vi "五参数水样测试.vi"(11 "启动参数":T1={"测量模式"=enum."水样测试", "数据标记表"="N", "测量时间"=3.0}) -> ()   [LabVIEW 2016, in "斯坦道仪器.lvlib"]
uses:
  PLC/PLC.lvlib
panel:
  out "枚举":T2(ring)
  out "状态":string
  out "数值":i32
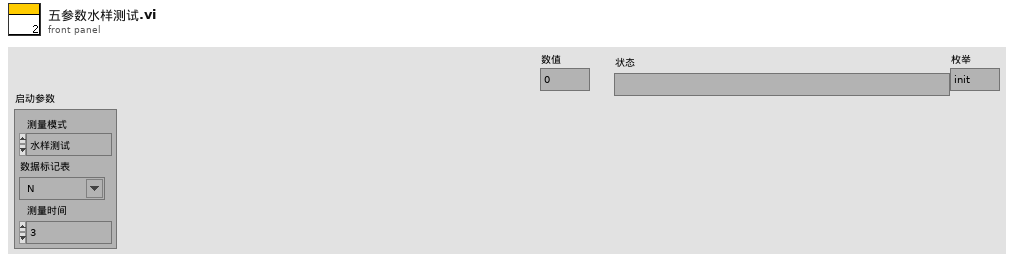
[diagram p1: front panel]
types:
  T1 = cluster{"测量模式":enum16{"待机", "水样测试", "标样核查", "零点核查", "跨度核查", "空白测试", "平行样测试", "加标回收", "空白校准", "标样校准", "初始化（清洗）"}, "数据标记表":string, "测量时间":dbl}
  T2 = enum16{"init", "开机", "启动测量", "读取测量值", "存储数据", "关闭测量", "关机", "结束"}
  T3 = cluster{"时间标识":timestamp, "设备":string, "日志信息":string, "流程参数":string}
  T4 = cluster{"starting address":u16, "holding register value":u16}
  T5 = enum16{"idle", "init", "读状态", "读参数", "多个写入", "单个写入", "线圈写入"}
  T6 = enum16{"待机", "水样测试", "标样核查", "零点核查", "跨度核查", "空白测试", "平行样测试", "加标回收", "空白校准", "标样校准", "初始化（清洗）"}
  T7 = cluster{"水温":dbl, "pH":dbl, "DO":dbl, "Cond":dbl, "Turb":dbl, "叶绿素":dbl, "藻密度":dbl, "蓝绿藻":dbl, "ORP":dbl, "NH3N":dbl}
  T8 = cluster{"数据标记表":string, "测量模式":enum16{"待机", "水样测试", "标样核查", "零点核查", "跨度核查", "空白测试", "平行样测试", "加标回收", "空白校准", "标样校准", "初始化（清洗）"}, "database":string}
  T9 = cluster{"因子编码":string, "单位":string, "标样参考值":sgl, "水样数据时间":timestamp, "水样实测值":sgl, "水样数据标识":string, "K":sgl, "B":sgl, "T":sgl, "H":sgl, "水深":sgl}
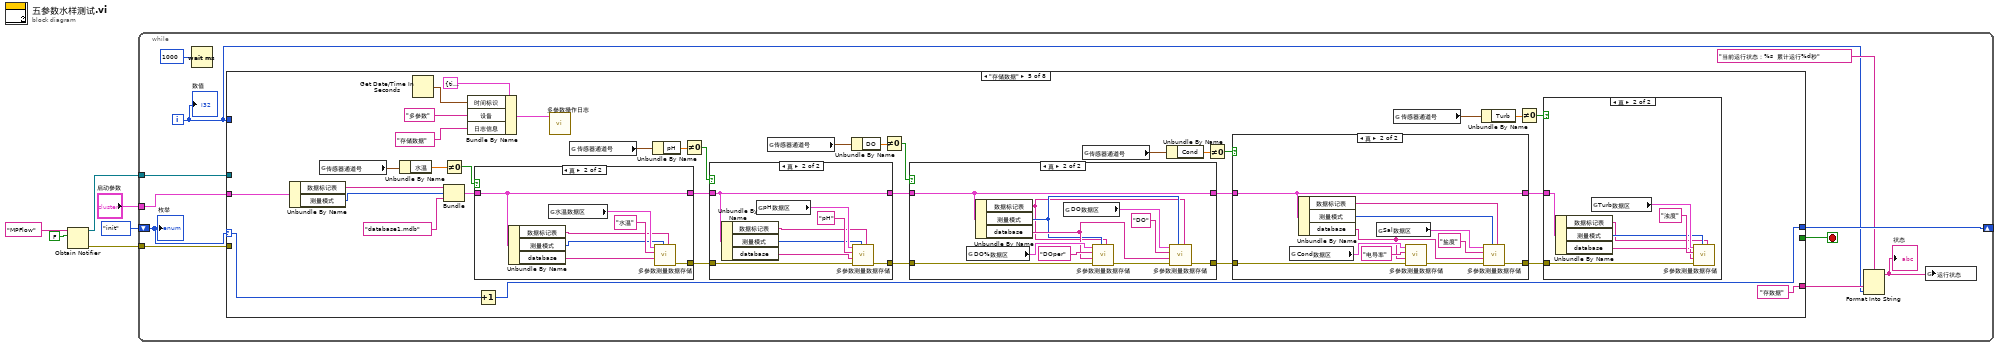
[diagram p0: block diagram]
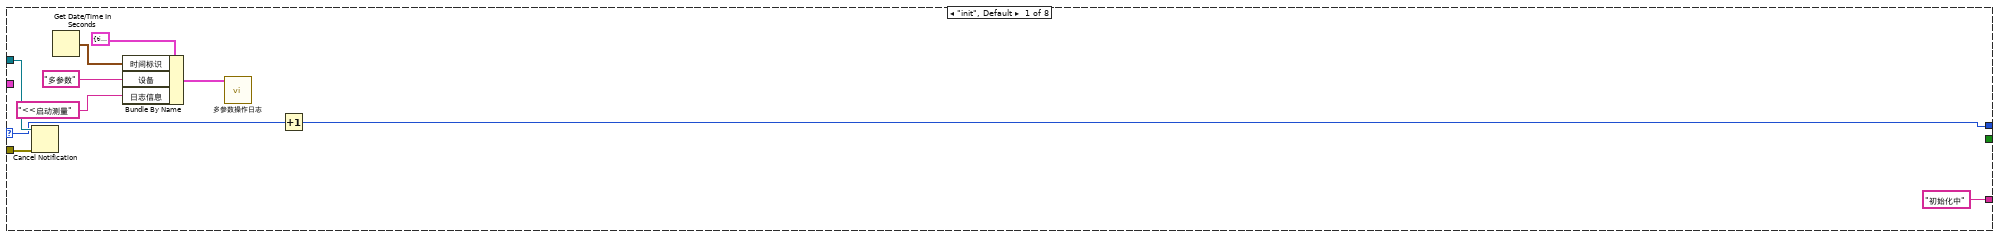
[diagram p2: hidden frame]
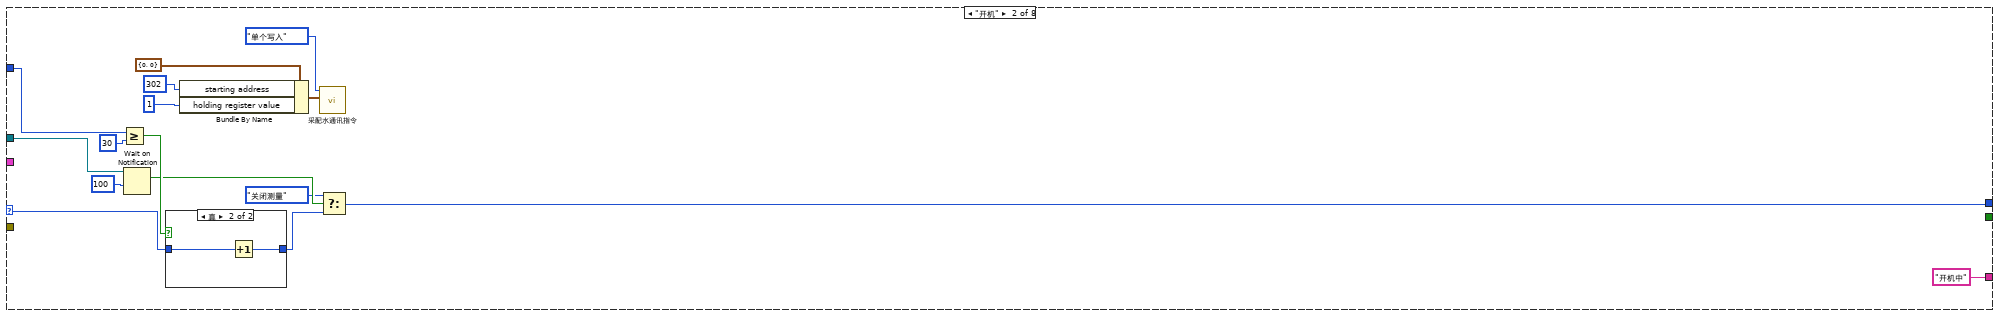
[diagram p3: hidden frame]
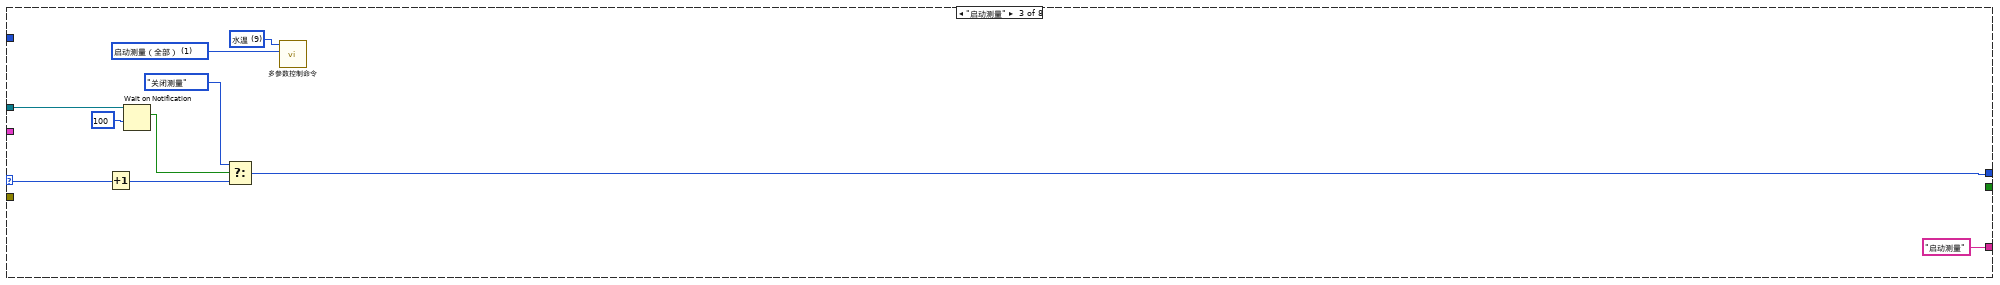
[diagram p5: hidden frame]
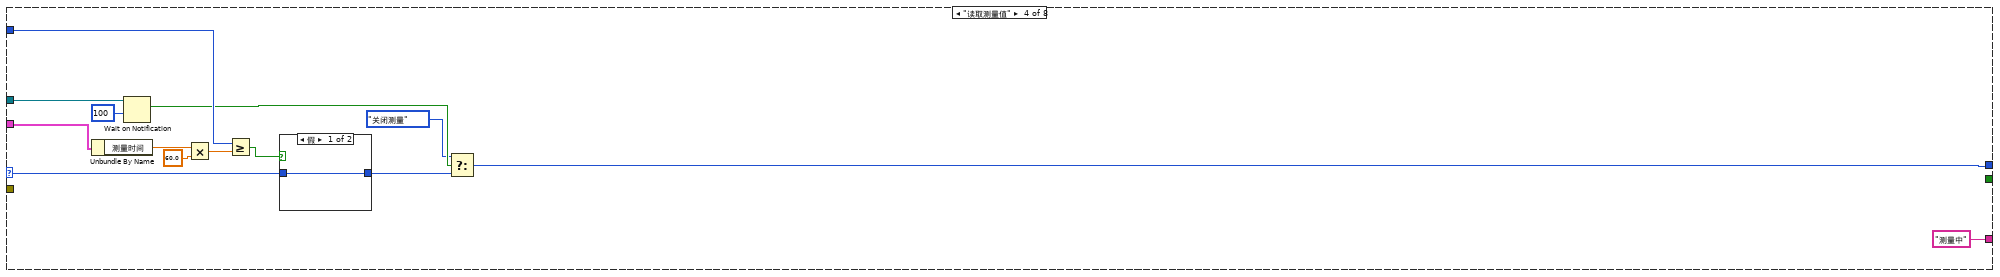
[diagram p6: hidden frame]
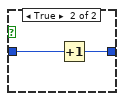
[diagram p7: hidden frame]
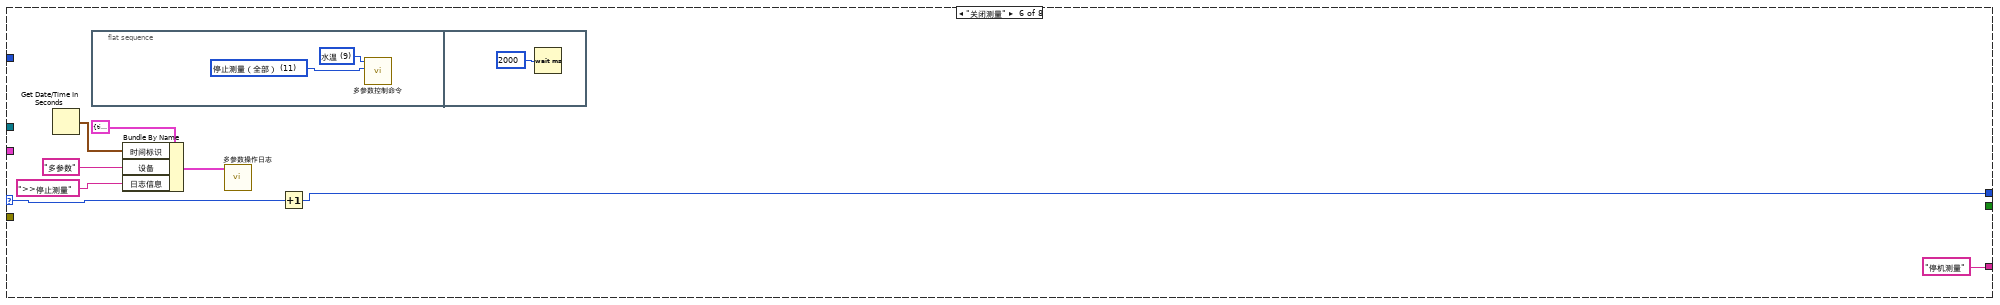
[diagram p13: hidden frame]
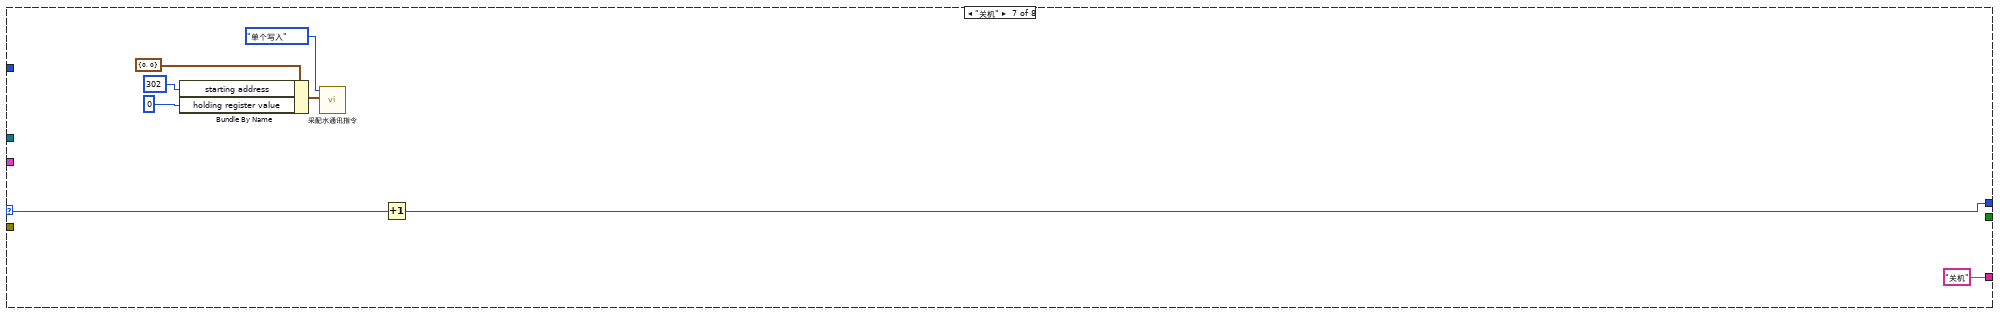
[diagram p14: hidden frame]
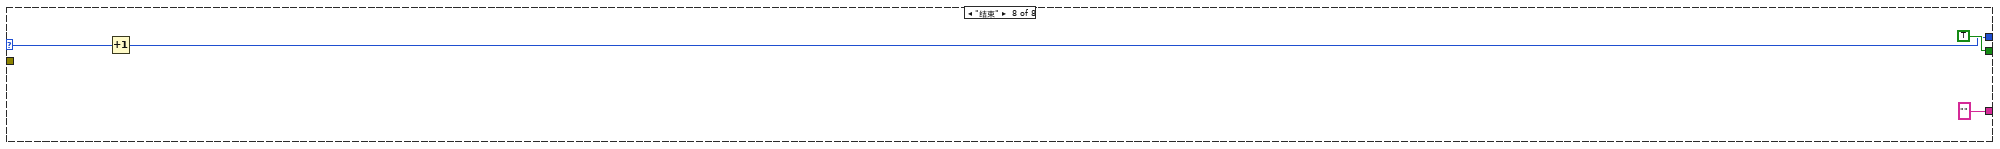
[diagram p15: hidden frame]
diagram:
  n1 = Obtain Notifier(name (unnamed)="MPFlow" ("名称（未命名）"), notification data type=FALSE) -> (notifier out=w3:refnum<notifier>, error out=w2:errorcluster)  [unwired: 2 in, 1 out]
  n2 = while {
    shift-right: [w13] -> _
    shift-left: T2."init" ("枚举") -> [w17]
    tunnel: w3 -> [w15]
    tunnel: w2 -> [w14]
    tunnel: "启动参数" -> [w7]
    i -> [w9]
    stop <- w16 stop-if-true
    n3 = Wait (ms)(milliseconds to wait=u32 1000 ("等待时间（毫秒）")) -> ()  [unwired: 1 out]
    n4 = case shown="\"存储数据\"" w17 {
      selector: w17 -> [w25 w38 w56 w69 w109 w165 w171 w179]
      tunnel: [_ _ _ _ _ _ _ TRUE] -> w16
      tunnel: w15 -> [w27 w33 w55 w66 _ _ _ _]
      tunnel: w14 -> [w26 _ _ _ _ _ _ _]
      tunnel: [w24 w31 w52 w64 w108 w164 w170 w178] -> w13
      tunnel: w9 -> [_ w37 _ w70 _ _ _ _]
      tunnel: ["初始化中" ("状态") "开机中" ("状态") "启动测量" ("状态") "测量中" ("状态") "存数据" ("状态") "停机测量" ("状态") "关机" ("状态") "" ("状态")] -> w10
      tunnel: w7 -> [_ _ _ w60 w106 _ _ _]
      frame "init", Default {
        n5 = Cancel Notification(0:w27, 3:w26) -> ()  [unwired: 3 out]
        n6 = Get Date/Time In Seconds() -> (seconds since 1Jan1904=w21:timestamp)
        n7 = Bundle By Name(cluster=T3 {"时间标识"=timestamp(0 s since 1904-01-01), "设备"="", "日志信息"="", "流程参数"=""} ("data in"), "时间标识"=w21, "设备"="多参数", "日志信息"="<<启动测量") -> (w20:T3)
        n8 = call "多参数操作日志.vi"("data in"=w20) -> ()  [unwired: 10 in, 1 out]
        n9 = Increment(x=w25) -> (x+1=w24:T2)
      }
      frame "开机" {
        n10 = Greater Or Equal?(x=w37, y=30) -> (x >= y?=w35:bool)
        n11 = Wait on Notification(notifier=w33, timeout in ms (-1)=100 ("超时毫秒(-1)")) -> (notification=w34:bool)  [unwired: 2 in, 3 out]
        n12 = case shown="真" w35 {
          tunnel: w38 -> [w44 w46]
          tunnel: [w44 w45] -> w32
          frame False {
          }
          frame True {
            n13 = Increment(x=w46) -> (x+1=w45:T2)
          }
        }
        n14 = Bundle By Name(cluster=T4 {"starting address"=0, "holding register value"=0}, "starting address"=u16 302, "holding register value"=u16 1) -> (w41:T4)
        n15 = call "采配水通讯指令.vi"("数据"=w41, "命令"=T5."单个写入") -> ()  [unwired: 10 in]
        n16 = Select(t=T2."关闭测量" ("枚举"), s=w34, f=w32) -> (s? t:f=w31:T2)
      }
      frame "启动测量" {
        w47 = u16 1 items=["启动测量（全部）"=1, "初始化（清洗）"=10, "停止测量（全部）"=11, "校时"=13, "启动测量（单个传感器）"=19, "停止测量（单个传感器）"=20] ("控制命令")
        w48 = u16 9 items=["氨氮"=3, "水温"=9, "pH值"=10, "溶解氧"=11, "电导率"=12, "浊度"=13, "叶绿素a"=14, "藻密度"=15, "蓝绿藻"=16, "氧化还原电位"=17, "溶解氧%"=18, "盐度"=19] ("站号")
        n17 = Increment(x=w56) -> (x+1=w53:T2)
        n18 = Wait on Notification(notifier=w55, timeout in ms (-1)=100 ("超时毫秒(-1)")) -> (notification=w54:bool)  [unwired: 2 in, 3 out]
        n19 = Select(t=T2."关闭测量" ("枚举"), s=w54, f=w53) -> (s? t:f=w52:T2)
        n20 = call "多参数控制命令.vi"("控制命令"=w47, "站号"=w48) -> ()  [unwired: 9 in, 1 out]
      }
      frame "读取测量值" {
        n21 = Unbundle By Name(w60) -> ("测量时间"=w59:dbl)
        n22 = Wait on Notification(notifier=w66, timeout in ms (-1)=100 ("超时毫秒(-1)")) -> (notification=w67:bool)  [unwired: 2 in, 3 out]
        n23 = Multiply(x=w59, y=60.0) -> (x*y=w57:dbl)
        n24 = Greater Or Equal?(x=w70, y=w57) -> (x >= y?=w68:bool)
        n25 = case shown="假" w68 {
          tunnel: w69 -> [w71 w73]
          tunnel: [w71 w72] -> w65
          frame False {
          }
          frame True {
            n26 = Increment(x=w73) -> (x+1=w72:T2)
          }
        }
        n27 = Select(t=T2."关闭测量" ("枚举"), s=w67, f=w65) -> (s? t:f=w64:T2)
      }
      frame "存储数据" {
        n28 = Unbundle By Name(w106) -> ("数据标记表"=w85:string, "测量模式"=w84:T6)
        n29 = global read "多参数全局变量.vi" "传感器通道号"() -> (w101:T7)
        n30 = Unbundle By Name(w101) -> ("水温"=w100:dbl)
        n31 = Get Date/Time In Seconds() -> (seconds since 1Jan1904=w77:timestamp)
        n32 = Not Equal To 0?(x=w100) -> (x != 0?=w99:bool)
        n33 = Bundle("数据标记表"=w85, "测量模式"=w84, "database"="database1.mdb") -> (w83:T8)  [unwired: 1 in]
        n34 = Bundle By Name(cluster=T3 {"时间标识"=timestamp(0 s since 1904-01-01), "设备"="", "日志信息"="", "流程参数"=""} ("data in"), "时间标识"=w77, "设备"="多参数", "日志信息"="存储数据") -> (w76:T3)
        n35 = case shown="真" w99 {
          tunnel: [_ w155] -> w105
          tunnel: w83 -> [w150 w154]
          tunnel: [w150 w154] -> w82
          frame False {
          }
          frame True {
            n36 = Unbundle By Name(w154) -> ("数据标记表"=w153:string, "测量模式"=w152:T6, "database"=w151:string)
            n37 = global read "多参数全局变量.vi" "水温数据区"() -> (w157:T9)
            n38 = call "多参数测量数据存储.vi"("数据标记表"=w153, "测量模式"=w152, "database"=w151, "table输入"="水温", "data in"=w157) -> ("error out"=w155:errorcluster)  [unwired: 6 in]
          }
        }
        n39 = Increment(x=w109) -> (x+1=w108:T2)
        n40 = call "多参数操作日志.vi"("data in"=w76) -> ()  [unwired: 10 in, 1 out]
        n41 = global read "多参数全局变量.vi" "传感器通道号"() -> (w94:T7)
        n42 = Unbundle By Name(w94) -> ("pH"=w93:dbl)
        n43 = Not Equal To 0?(x=w93) -> (x != 0?=w98:bool)
        n44 = case shown="真" w98 {
          tunnel: w105 -> [_ w149]
          tunnel: [_ w147] -> w104
          tunnel: w82 -> [w141 w145]
          tunnel: [w141 w145] -> w80
          frame False {
          }
          frame True {
            n45 = Unbundle By Name(w145) -> ("数据标记表"=w144:string, "测量模式"=w143:T6, "database"=w142:string)
            n46 = global read "多参数全局变量.vi" "pH数据区"() -> (w148:T9)
            n47 = call "多参数测量数据存储.vi"("数据标记表"=w144, "测量模式"=w143, "error in (no error)"=w149, "database"=w142, "table输入"="pH", "data in"=w148) -> ("error out"=w147:errorcluster)  [unwired: 5 in]
          }
        }
        n48 = global read "多参数全局变量.vi" "传感器通道号"() -> (w92:T7)
        n49 = Unbundle By Name(w92) -> ("DO"=w91:dbl)
        n50 = Not Equal To 0?(x=w91) -> (x != 0?=w97:bool)
        n51 = case shown="真" w97 {
          tunnel: w104 -> [_ w140]
          tunnel: [_ w136] -> w103
          tunnel: [w129 w133] -> w81
          tunnel: w80 -> [w129 w133]
          frame False {
          }
          frame True {
            n52 = global read "多参数全局变量.vi" "DO%数据区"() -> (w135:T9)
            n53 = Unbundle By Name(w133) -> ("数据标记表"=w130:string, "测量模式"=w131:T6, "database"=w132:string)
            n54 = global read "多参数全局变量.vi" "DO数据区"() -> (w137:T9)
            n55 = call "多参数测量数据存储.vi"("数据标记表"=w130, "测量模式"=w131, "error in (no error)"=w140, "database"=w132, "table输入"="DOper", "data in"=w135) -> ("error out"=w139:errorcluster)  [unwired: 5 in]
            n56 = call "多参数测量数据存储.vi"("数据标记表"=w130, "测量模式"=w131, "error in (no error)"=w139, "database"=w132, "table输入"="DO", "data in"=w137) -> ("error out"=w136:errorcluster)  [unwired: 5 in]
          }
        }
        n57 = global read "多参数全局变量.vi" "传感器通道号"() -> (w90:T7)
        n58 = Unbundle By Name(w90) -> ("Cond"=w89:dbl)
        n59 = Not Equal To 0?(x=w89) -> (x != 0?=w96:bool)
        n60 = case shown="真" w96 {
          tunnel: w103 -> [_ w126]
          tunnel: [_ w122] -> w102
          tunnel: w81 -> [w117 w121]
          tunnel: [w117 w121] -> w79
          frame False {
          }
          frame True {
            n61 = global read "多参数全局变量.vi" "Cond数据区"() -> (w128:T9)
            n62 = Unbundle By Name(w121) -> ("数据标记表"=w118:string, "测量模式"=w119:T6, "database"=w120:string)
            n63 = global read "多参数全局变量.vi" "Sal数据区"() -> (w124:T9)
            n64 = call "多参数测量数据存储.vi"("error in (no error)"=w126, "database"=w120, "table输入"="电导率", "data in"=w128) -> ("error out"=w125:errorcluster)  [unwired: 7 in]
            n65 = call "多参数测量数据存储.vi"("数据标记表"=w118, "测量模式"=w119, "error in (no error)"=w125, "database"=w120, "table输入"="盐度", "data in"=w124) -> ("error out"=w122:errorcluster)  [unwired: 5 in]
          }
        }
        n66 = global read "多参数全局变量.vi" "传感器通道号"() -> (w88:T7)
        n67 = Unbundle By Name(w88) -> ("Turb"=w87:dbl)
        n68 = Not Equal To 0?(x=w87) -> (x != 0?=w95:bool)
        n69 = case shown="真" w95 {
          tunnel: w102 -> [_ w116]
          tunnel: w79 -> [_ w113]
          frame False {
          }
          frame True {
            n70 = Unbundle By Name(w113) -> ("数据标记表"=w110:string, "测量模式"=w111:T6, "database"=w112:string)
            n71 = global read "多参数全局变量.vi" "Turb数据区"() -> (w115:T9)
            n72 = call "多参数测量数据存储.vi"("数据标记表"=w110, "测量模式"=w111, "error in (no error)"=w116, "database"=w112, "table输入"="浊度", "data in"=w115) -> ()  [unwired: 5 in, 1 out]
          }
        }
      }
      frame "关闭测量" {
        n73 = Get Date/Time In Seconds() -> (seconds since 1Jan1904=w161:timestamp)
        n74 = flat-sequence {
          frame #0 {
            w166 = u16 11 items=["启动测量（全部）"=1, "初始化（清洗）"=10, "停止测量（全部）"=11, "校时"=13, "启动测量（单个传感器）"=19, "停止测量（单个传感器）"=20] ("控制命令")
            w167 = u16 9 items=["氨氮"=3, "水温"=9, "pH值"=10, "溶解氧"=11, "电导率"=12, "浊度"=13, "叶绿素a"=14, "藻密度"=15, "蓝绿藻"=16, "氧化还原电位"=17, "溶解氧%"=18, "盐度"=19] ("站号")
            n75 = call "多参数控制命令.vi"("控制命令"=w166, "站号"=w167) -> ()  [unwired: 9 in, 1 out]
          }
          frame #1 {
            n76 = Wait (ms)(milliseconds to wait=u32 2000 ("等待时间（毫秒）")) -> ()  [unwired: 1 out]
          }
        }
        n77 = Bundle By Name(cluster=T3 {"时间标识"=timestamp(0 s since 1904-01-01), "设备"="", "日志信息"="", "流程参数"=""} ("data in"), "时间标识"=w161, "设备"="多参数", "日志信息"=">>停止测量") -> (w160:T3)
        n78 = call "多参数操作日志.vi"("data in"=w160) -> ()  [unwired: 10 in, 1 out]
        n79 = Increment(x=w165) -> (x+1=w164:T2)
      }
      frame "关机" {
        n80 = Bundle By Name(cluster=T4 {"starting address"=0, "holding register value"=0}, "starting address"=u16 302, "holding register value"=u16 0) -> (w174:T4)
        n81 = call "采配水通讯指令.vi"("数据"=w174, "命令"=T5."单个写入") -> ()  [unwired: 10 in]
        n82 = Increment(x=w171) -> (x+1=w170:T2)
      }
      frame "结束" {
        n83 = Increment(x=w179) -> (x+1=w178:T2)
      }
    }
    n84 = Format Into String(format string="当前运行状态：%s  累计运行%d秒" ("格式字符串"), w10, w9) -> (resulting string=w8:string)  [unwired: 2 in, 1 out]
    "状态" <- w8
    n85 = global write "多参数全局变量.vi" "运行状态"(w8) -> ()
    "数值" <- w9
    "枚举" <- w17
  }
